vi "Get targets.vi"(8 "error in (no error)":errorcluster, 9 "Ramp rate (T/min)":dbl, 10 "Setpoint (T)":dbl, 11 "CurrentToField in":refnum<class "CurrentToField.lvclass">) -> (0 "error out":errorcluster, 1 "Ramp rates (A/s)":T2, 2 "Setpoints (A)":T3, 3 "CurrentToField out":refnum<class "CurrentToField.lvclass">, 4 "Coerced Inputs":T1)   [LabVIEW 2024, in "CurrentToField.lvclass"]
uses:
  CurrentToField.lvclass
  CurrentToField.lvclass/CurrentToField.ctl
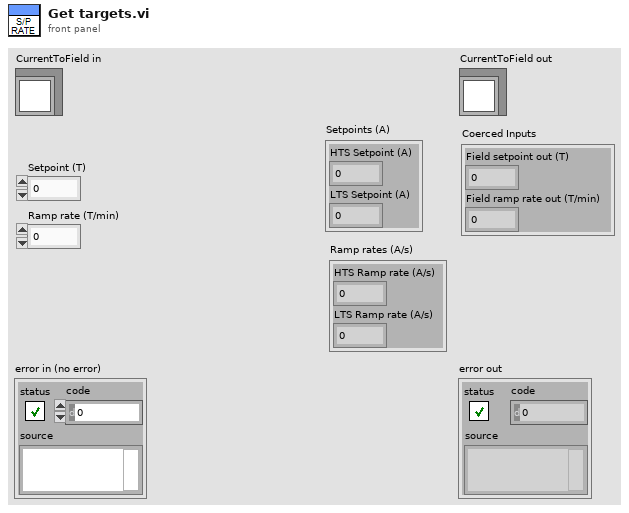
[diagram p1: front panel]
types:
  T1 = cluster{"Field setpoint out (T)":dbl, "Field ramp rate out (T/min)":dbl}
  T2 = cluster{"HTS Ramp rate (A/s)":dbl, "LTS Ramp rate (A/s)":dbl}
  T3 = cluster{"HTS Setpoint (A)":dbl, "LTS Setpoint (A)":dbl}
  T4 = cluster{"Setpoint (T)":dbl, "Max combined rate (T/min)":dbl}
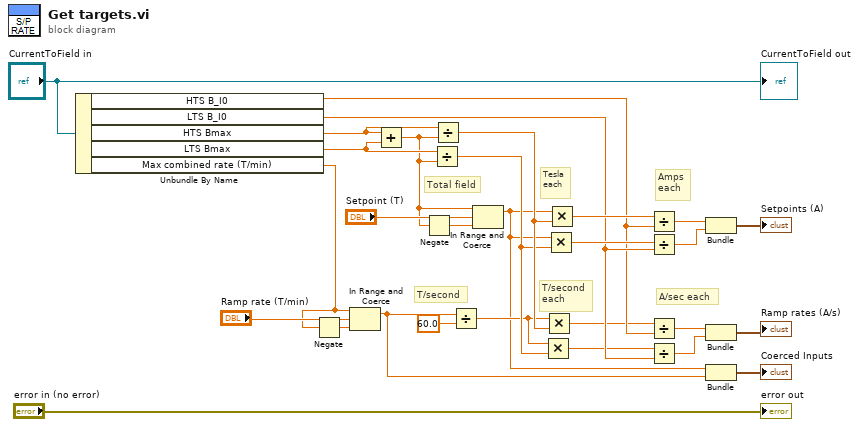
[diagram p0: block diagram]
diagram:
  # "Total field"
  # "A/sec each"
  # "T/second\neach"
  # "T/second"
  # "Amps\neach"
  # "Tesla\neach"
  n1 = Unbundle By Name("CurrentToField in") -> ("HTS B_I0"=w19:dbl, "LTS B_I0"=w20:dbl, "HTS Bmax"=w26:dbl, "LTS Bmax"=w27:dbl, "Max combined rate (T/min)"=w10:dbl)
  n2 = Negate(x=w10) -> (-x=w11:dbl)
  n3 = In Range and Coerce(upper limit=w10, x="Ramp rate (T/min)", lower limit=w11) -> (coerced(x)=w8:dbl)  [unwired: 1 out]
  n4 = Add(x=w26, y=w27) -> (x+y=w14:dbl)
  n5 = Negate(x=w14) -> (-x=w15:dbl)
  n6 = Divide(x=w27, y=w14) -> (x/y=w21:dbl)
  n7 = Divide(x=w26, y=w14) -> (x/y=w22:dbl)
  n8 = Divide(x=w8, y=60.0) -> (x/y=w13:dbl)
  n9 = In Range and Coerce(upper limit=w14, x="Setpoint (T)", lower limit=w15) -> (coerced(x)=w9:dbl)  [unwired: 1 out]
  n10 = Multiply(x=w13, y=w21) -> (x*y=w17:dbl)
  n11 = Multiply(x=w13, y=w22) -> (x*y=w18:dbl)
  n12 = Multiply(x=w9, y=w21) -> (x*y=w25:dbl)
  n13 = Multiply(x=w9, y=w22) -> (x*y=w24:dbl)
  n14 = Divide(x=w24, y=w19) -> (x/y=w2:dbl)
  n15 = Divide(x=w25, y=w20) -> (x/y=w1:dbl)
  n16 = Divide(x=w18, y=w19) -> (x/y=w6:dbl)
  n17 = Divide(x=w17, y=w20) -> (x/y=w5:dbl)
  n18 = Bundle(w2, w1) -> (→"Setpoints (A)":cluster{dbl, dbl})  [unwired: 1 in]
  n19 = Bundle(w6, w5) -> (→"Ramp rates (A/s)":cluster{dbl, dbl})  [unwired: 1 in]
  n20 = Bundle("Setpoint (T)"=w9, "Max combined rate (T/min)"=w8) -> (→"Coerced Inputs":T4)  [unwired: 1 in]
  "error out" <- "error in (no error)"
  "CurrentToField out" <- "CurrentToField in"
